vi "Construct Configuration Object.vi"(6 "Group Name":string, 7 "Window Title":string, 8 "error in (no error)":errorcluster, 9 "Initial Category Selection":i32=-1, 10 "Configuration File Path":path, 11 "Configuration in":refnum<class "Configuration.lvclass">) -> (0 "error out":errorcluster, 1 "Stop Event":refnum<user-event>, 2 "Path to config file":path, 3 "Configuration out":refnum<class "Configuration.lvclass">)   [LabVIEW 2020, in "Configuration.lvlib" / "Configuration.lvclass"]
uses:
  Configuration.lvclass
  <vilib>/Utility/sysdir.llb/System Directory Type.ctl
  Configuration.lvclass/Configuration.ctl
  <userlib>/_OpenG.lib/file/file.llb/Valid Path - Traditional__ogtk.vi
  <userlib>/_OpenG.lib/file/file.llb/File Exists - Scalar__ogtk.vi
  <userlib>/_OpenG.lib/file/file.llb/Convert File Extension (Path)__ogtk.vi
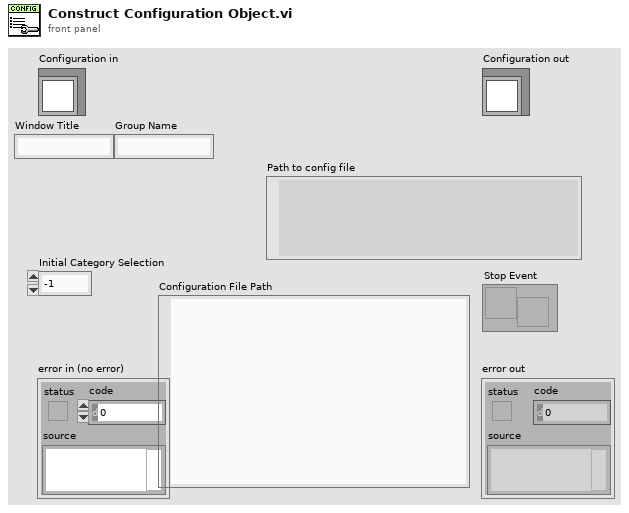
[diagram p1: front panel]
types:
  T1 = typedef "System Directory Type.ctl" = i32
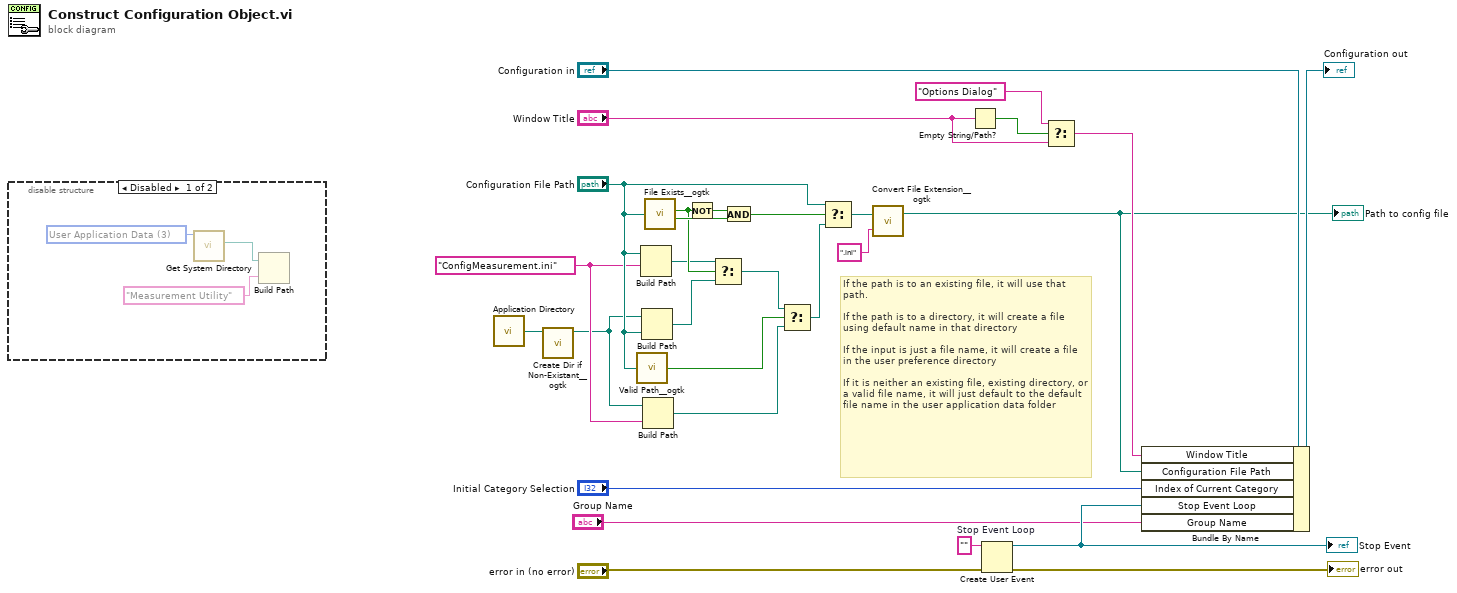
[diagram p0: block diagram]
diagram:
  w11 = "ConfigMeasurement.ini" ("name or relative path")
  w26 = ""  # Stop Event Loop
  # "If the path is to an existing file, it will use that path.\n\nIf the path is to a directory, it will create a file using default name in that directory\n\nIf the input is just a file name, it will create a file in the user preference directory\n\nIf it is neither an existing file, existing directory, or a valid file name, it will just default to the default file name in the user application data folder"
  n1 = disable-structure shown="Disabled" {
    frame Disabled {
      w32 = T1 3 items=["User Home"=0, "User Desktop"=1, "User Documents"=2, "User Application Data"=3, "User Preferences"=4, "User Temporary"=5, "Public Documents"=6, "Public Application Data"=7, "Public Preferences"=8, "Public Cache"=13, "System Core Libraries"=9, "System Installed Libraries"=10, "Application Files"=11, "Boot Volume Root"=12] ("system directory type")
      n2 = call <vilib>:"Get System Directory.vi"("system directory type"=w32) -> ("system directory"=w30:path)  [unwired: 10 in]
      n3 = Build Path(base path=w30, name or relative path="Measurement Utility") -> ()  [unwired: 1 out]
    }
    frame Enabled {
    }
  }
  n4 = call <vilib>:"Application Directory.vi"() -> ("Application Directory"=w1:path)
  n5 = call <userlib>:"Create Dir if Non-Existant__ogtk.vi"("Directory Path"=w1) -> ("dup Directory Path"=w3:path)  [unwired: 8 in, 2 out]
  n6 = call-poly <userlib>:"Valid Path__ogtk.vi"("path"="Configuration File Path") -> ("valid"=w10:bool)
  n7 = Build Path(base path="Configuration File Path", name or relative path=w11) -> (appended path=w14:path)
  n8 = Build Path(base path=w3, name or relative path="Configuration File Path") -> (appended path=w13:path)
  n9 = Build Path(base path=w3, name or relative path=w11) -> (appended path=w9:path)
  n10 = call-poly <userlib>:"File Exists__ogtk.vi"("file path"="Configuration File Path") -> ("is directory"=w15:bool, "exists"=w17:bool)  [unwired: 6 in]
  n11 = Not(x=w15) -> (.not. x?=w18:bool)
  n12 = Select(t=w14, s=w15, f=w13) -> (s? t:f=w8:path)
  n13 = And(x=w18, y=w17) -> (x .and. y?=w16:bool)
  n14 = Select(t=w8, s=w10, f=w9) -> (s? t:f=w7:path)
  n15 = Select(t="Configuration File Path", s=w16, f=w7) -> (s? t:f=w6:path)
  n16 = call-poly <userlib>:"Convert File Extension__ogtk.vi"("new ending (none)"=".ini" ("y"), "file name"=w6) -> ("new filename"=w4:path)  [unwired: 1 out]
  "Path to config file" <- w4
  n17 = Empty String/Path?(string/path="Window Title") -> (empty?=w23:bool)
  n18 = Create User Event(user event datatype=w26, error in="error in (no error)") -> (user event=w27:refnum<user-event>, error out=→"error out":errorcluster)
  "Stop Event" <- w27
  n19 = Select(t="Options Dialog" ("Window Title"), s=w23, f="Window Title") -> (s? t:f=w20:string)
  n20 = Bundle By Name(cluster="Configuration in", "Window Title"=w20, "Configuration File Path"=w4, "Index of Current Category"="Initial Category Selection", "Stop Event Loop"=w27, "Group Name"="Group Name") -> (→"Configuration out":refnum<class "Configuration.lvclass">)
